vi "Set Switch Heater.vi"(8 "error in (no error)":errorcluster, 10 "Switch Heater":T1, 11 "Instrument.1820 in":refnum<class "Instrument.Oxford1820.lvclass">) -> (0 "error out":errorcluster, 3 "Instrument.1820 in":refnum<class "Instrument.Oxford1820.lvclass">)   [LabVIEW 2016, in "Instrument.Oxford1820.lvclass"]
uses:
  Instrument.Oxford1820.lvclass
  <instrlib>/Mercury iXX/Public/Libraries/Magnet/Controls/Switch Heater.ctl
  Typedefs/Instrument.Oxford1820.Commands-enum.ctl
  <instrlib>/Mercury iXX/Public/Libraries/Magnet.lvlib
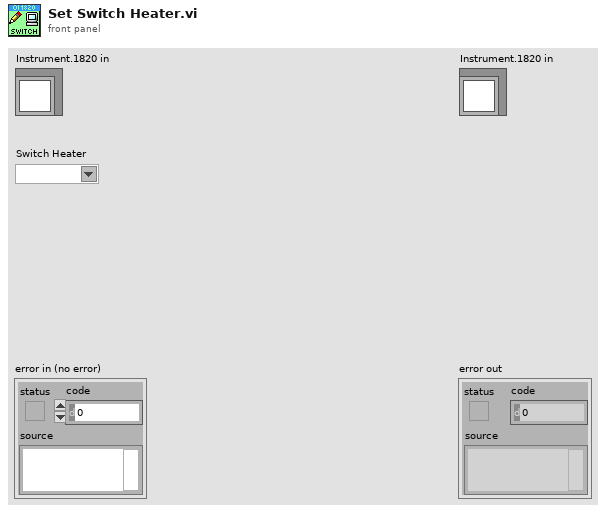
[diagram p1: front panel]
types:
  T1 = typedef "Mercury iXX.lvlib/Magnet.lvlib/Switch Heater.ctl" = string
  T2 = typedef "Instrument.Oxford1820.lvclass/Instrument.Oxford1820.Commands-enum.ctl" = enum16{"setAction", "setTarget", "setSwitchHeat", "setLambda", "setFillMode", "setNeedleValve", "setMagnetField", "getStatus", "getTarget", "getSwitchHeat", "getPSUField", "getMagnetField"}
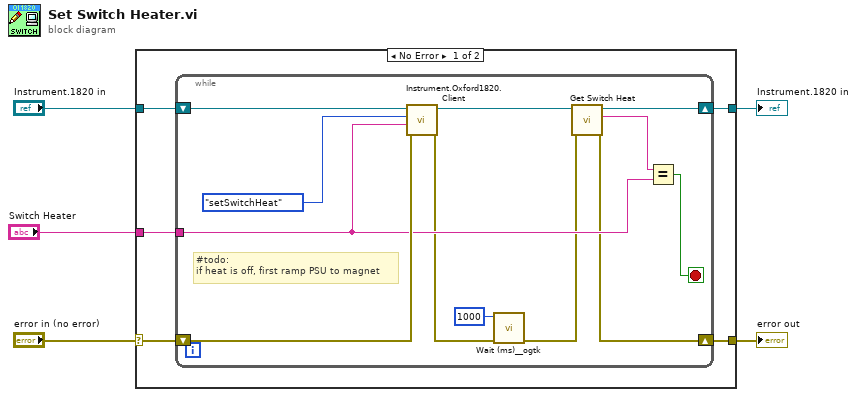
[diagram p0: block diagram]
diagram:
  n1 = case shown="No Error" "error in (no error)" {
    selector: "error in (no error)" -> [w9 w24]
    tunnel: [w8 w24] -> w4
    tunnel: [w7 w23] -> w2
    tunnel: "Instrument.1820 in" -> [w10 w23]
    tunnel: "Switch Heater" -> [w6 _]
    frame No Error {
      n2 = while {
        tunnel: w6 -> [w18]
        shift-right: [w20] -> w7
        shift-left: w10 -> [w12]
        shift-right: [w15] -> w8
        shift-left: w9 -> [w21]
        stop <- w17 stop-if-true
        # "#todo:\nif heat is off, first ramp PSU to magnet"
        n3 = call "Instrument.Oxford1820.Client.vi"("error in (no error)"=w21, "Data"=w18, "Commands"=Instrument.Oxford1820.Commands-enum."setSwitchHeat", "Instrument.1820 in"=w12) -> ("error out"=w16:errorcluster, "Instrument.1820 out"=w11:refnum<class "Instrument.Oxford1820.lvclass">)  [unwired: 5 in, 1 out]
        n4 = call <userlib>:"Wait (ms)__ogtk.vi"("error in (no error)"=w16, "milliseconds to wait"=u32 1000) -> ("error out"=w14:errorcluster)  [unwired: 8 in, 1 out]
        n5 = call "Get Switch Heat.vi"("error in (no error)"=w14, "Instrument.1820 in"=w11) -> ("error out"=w15:errorcluster, "Switch Heater Status"=w19:string, "Instrument.1820 in"=w20:refnum<class "Instrument.Oxford1820.lvclass">)  [unwired: 6 in, 1 out]
        n6 = Equal?(x=w19, y=w18) -> (x = y?=w17:bool)
      }
    }
    frame Error {
    }
  }
  "error out" <- w4
  "Instrument.1820 in" <- w2
